vi "DriveSubsystem.vi"   [LabVIEW 2017]
panel:
  # "This is responsable for drive train control"
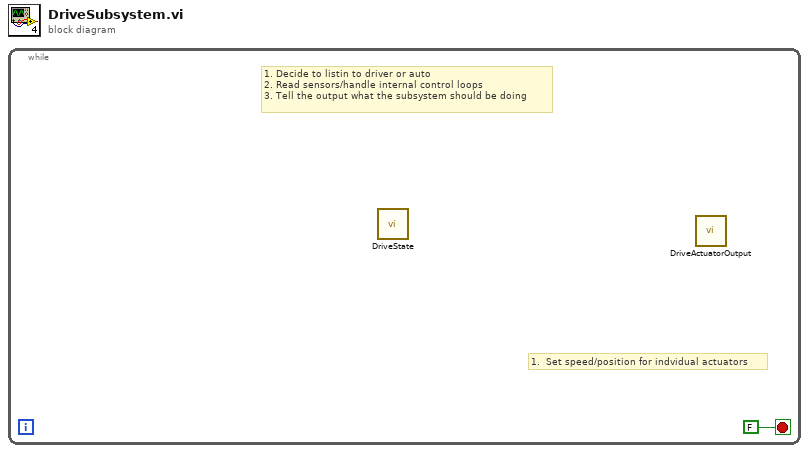
[diagram p0: block diagram]
diagram:
  n1 = while {
    stop <- FALSE stop-if-true
    # "1.  Set speed/position for indvidual actuators"
    # "1. Decide to listin to driver or auto\n2. Read sensors/handle internal control loops\n3. Tell the output what the subsystem should be doing"
    n2 = call "DriveState.vi"() -> ()  [unwired: 12 in]
    n3 = call "DriveActuatorOutput.vi"() -> ()  [unwired: 12 in]
  }
